vi "intensityChart.vi"() -> ()   [LabVIEW 2014]
uses:
  <vilib>/gmath/statdist.llb/Normal PDF.vi
  <vilib>/gmath/NI_Gmath.lvlib
panel:
  in  "Gaussian Parameters":T1 {"Mean" scale=0.0..200.0; "Std Dev." scale=1.0..50.0; "Normalization" scale=1.0..10.0}
  in  "Data Per Sample":i32(slide) scale=10.0..200.0
  in  "Stop Plotting":bool
  out "Intensity Chart":dbl[][](graph)
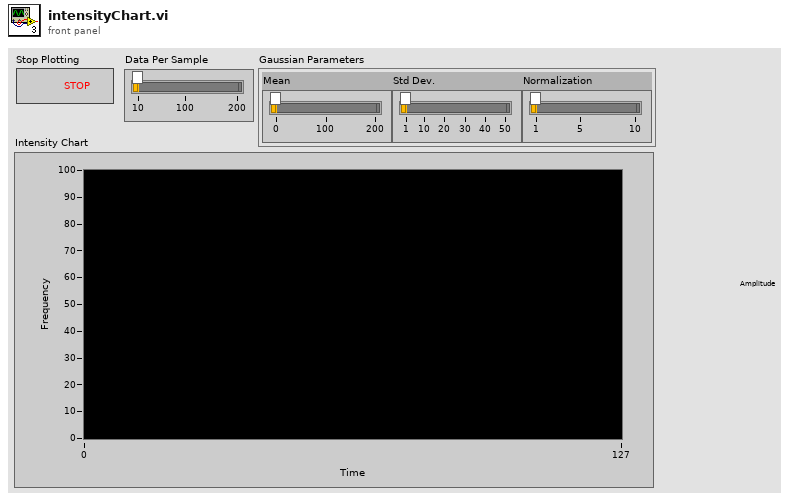
[diagram p1: front panel]
types:
  T1 = cluster{"Mean":dbl, "Std Dev.":dbl, "Normalization":dbl}
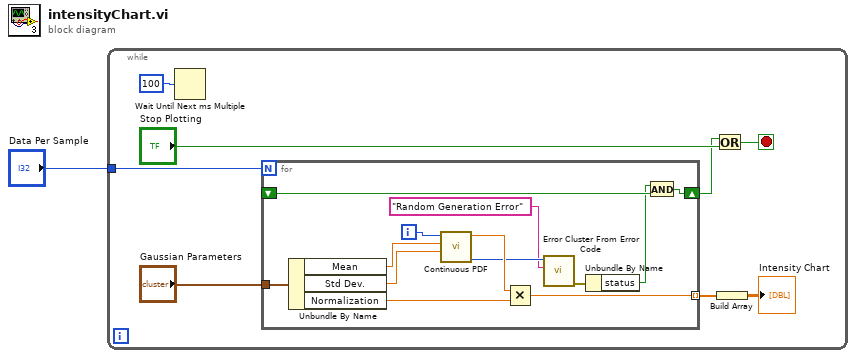
[diagram p0: block diagram]
diagram:
  n1 = while {
    tunnel: "Data Per Sample" -> [w8]
    stop <- w7 stop-if-true
    n2 = Wait Until Next ms Multiple(millisecond multiple=u32 100) -> ()  [unwired: 1 out]
    n3 = for {
      N: w8 -> [_]
      tunnel: [w15] -> w6 mode=indexing
      tunnel: "Gaussian Parameters" -> [w14]
      shift-right: [w10] -> w2
      shift-left: _ -> [w12]
      i -> [w22]
      n4 = Unbundle By Name(w14) -> ("Mean"=w21:dbl, "Std Dev."=w20:dbl, "Normalization"=w18:dbl)
      n5 = call-poly <vilib>:"Continuous PDF.vi"("std"=w20, "mean"=w21, "x"=w22) -> ("error"=w17:i32, "pdf(x)"=w19:dbl)  [unwired: 7 in]
      n6 = Multiply(x=w19, y=w18) -> (x*y=w15:dbl)
      n7 = call <vilib>:"Error Cluster From Error Code.vi"("error message (\"\")"="Random Generation Error" ("error message (\"\")"), "error code (0)"=w17) -> ("error out"=w13:errorcluster)  [unwired: 7 in]
      n8 = Unbundle By Name(w13) -> ("status"=w11:bool)
      n9 = And(x=w11, y=w12) -> (x .and. y?=w10:bool)
    }
    n10 = Or(x=w2, y="Stop Plotting") -> (x .or. y?=w7:bool)
    n11 = Build Array(w6) -> (→"Intensity Chart":dbl[][])
  }
